vi "export waveforms to spreadhseet with modified timestamps.vi"() -> ()   [LabVIEW 2016]
panel:
  in  "trial start time":timestamp
  in  "waveform":waveform(dbl)
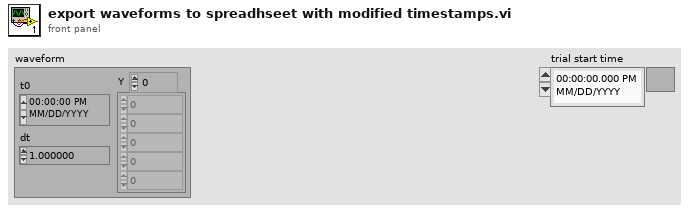
[diagram p1: front panel]
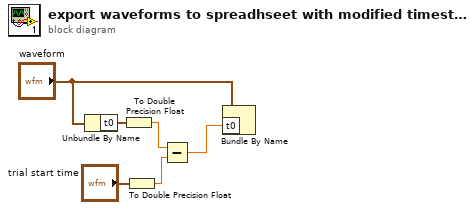
[diagram p0: block diagram]
diagram:
  n1 = Unbundle By Name("waveform") -> ("t0"=w4:timestamp)
  n2 = To Double Precision Float(number=w4) -> (double precision float=w3:dbl)
  n3 = To Double Precision Float(number="trial start time") -> (double precision float=w2:dbl)
  n4 = Subtract(x=w3, y=w2) -> (x-y=w1:dbl)
  n5 = Bundle By Name(cluster="waveform", "t0"=w1) -> ()  [unwired: 1 out]
